vi "lm Get LE State.vi"(8 "error in (no error)":errorcluster) -> (0 "error out":errorcluster, 3 "function return":i32)   [LabVIEW 2018, in "LumencorDLL32.lvlib"]
doc: "This function reads back the state of the Sola or SolaSE (Only) See DLL documentation for instructions on decoding returned value.\n\nextern \"C\" LUMENCORDLL2B_API int lmGetLEState(void);"
uses:
  LumencorDLL32.lvlib
  LumencorDLL32.dll
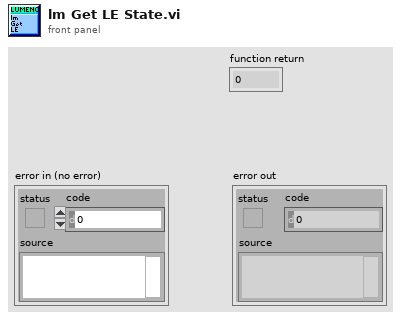
[diagram p1: front panel]
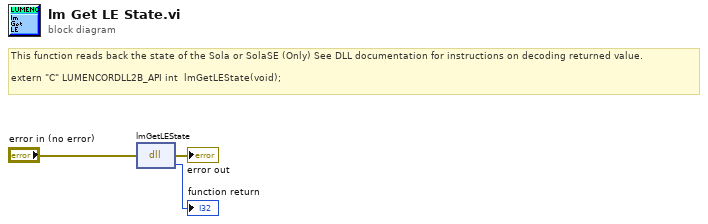
[diagram p0: block diagram]
diagram:
  # "This function reads back the state of the Sola or SolaSE (Only) See DLL documentation for instructions on decoding returned value.\n\nextern \"C\" LUMENCORDLL2B_API int  lmGetLEState(void);"
  n1 = dll-call lib="C:/Users/e14user/Documents/LabVIEW software/GitRepo/lib/SOLA/LabVIEW 2015 Library (32bit)/LumencorDLL32/LumencorDLL32.*" fn="lmGetLEState"(error in="error in (no error)") -> (error out=→"error out":errorcluster, →"function return":i32)  [unwired: 2 in, 1 out]
